vi "set_target_configuration.vi"(8 "error in":errorcluster, 10 "Target Configuration Data":T1, 11 "target ref":refnum<k24>) -> (0 "error out":errorcluster, 3 "target ref out":refnum<k24>)   [LabVIEW 2020]
uses:
  NationalInstruments.VeriStand.SystemDefinitionAPI
  controls/target_configuration_cluster.ctl
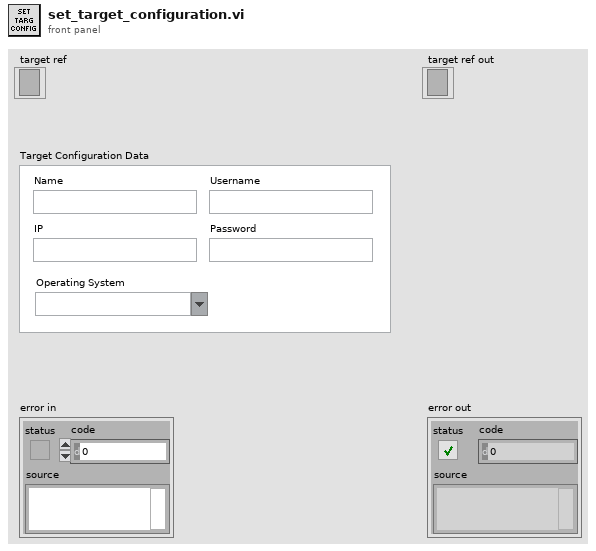
[diagram p1: front panel]
types:
  T1 = typedef "target_configuration_cluster.ctl" = cluster{"Name":string, "IP":string, "Username":string, "Password":string, "Operating System":string}
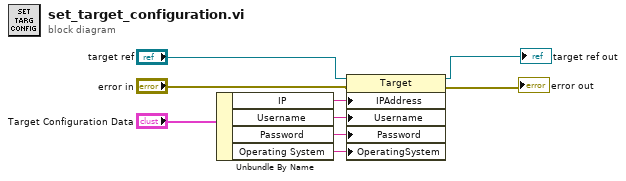
[diagram p0: block diagram]
diagram:
  n1 = Unbundle By Name("Target Configuration Data") -> ("IP"=w7:string, "Username"=w6:string, "Password"=w5:string, "Operating System"=w1:string)
  n2 = property class="Target"(reference="target ref", error in="error in", "IPAddress"=w7, "Username"=w6, "Password"=w5, "OperatingSystem"=w1) -> (reference out=→"target ref out":refnum<k24>, error out=→"error out":errorcluster)
